vi "ClientGlobal.vi"() -> ()   [LabVIEW 2014]
panel:
  in  "TimeDelay":u32=100
  out "Menu":refnum<k9>
  out "check array":u8[](array[numeric])
  out "PwdChecked?":bool
  out "UserName":string
  in  "connection ID":refnum<k5>
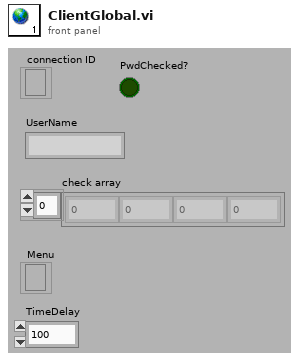
[diagram p1: front panel]
diagram:
